vi "Robot Global Data.vi"() -> ()   [LabVIEW 2017]
doc: "This global VI can contain as many global variables as you need. Place a control on the panel, give it a good name. To read or write to it from a VI, drag the icon to the diagram of that VI. You can also drag from the project. Click on the node to change which global you access. You shouldn't have multiple locations writing to a global or it will cause a race-condition."
uses:
  <vilib>/Rock Robotics/WPI/Camera/WPI_CameraImageSize.ctl
  <vilib>/Rock Robotics/WPI/DriverStation/WPI_DriverStationRobotMode2.ctl
panel:
  in  "MotionProfilePos_Right":dbl
  in  "MotionProfilePos_Left":dbl
  in  "Left Drive Position":dbl
  in  "Right Drive Position":dbl
  in  "AutoSwitch":bool
  in  "Record Auto?":bool
  in  "Left Drive Speed":dbl
  in  "Right Drive Speed":dbl
  in  "pistonLock":bool
  in  "MotionProfileVel_Right":dbl
  in  "MotionProfileVel_Left":dbl
  in  "rightEncoder":i32
  in  "leftEncoder":i32
  in  "desiredAngle":dbl
  out "resetEncoder":bool
  in  "distanceInCounts":dbl
  in  "driveStraightSpeed":dbl
  in  "navXYaw":dbl
  in  "leftButtons":bool[](array[boolean])
  in  "manualFirst":bool
  in  "2slide":dbl
  out "secondBottom":bool
  out "secondTop":bool
  out "firstBottom":bool
  out "firstTop":bool
  in  "clawOut":bool
  in  "clawIn":bool
  in  "clawOpen":bool
  in  "clawUp":bool
  in  "driveModes":T1(ring)
  out "rightDrivePower":dbl
  out "leftDrivePower":dbl
  in  "1Sslide":dbl
  in  "Robot Mode":T2
  in  "image size":T3=enum."320x240"
  in  "Enable Vision":bool
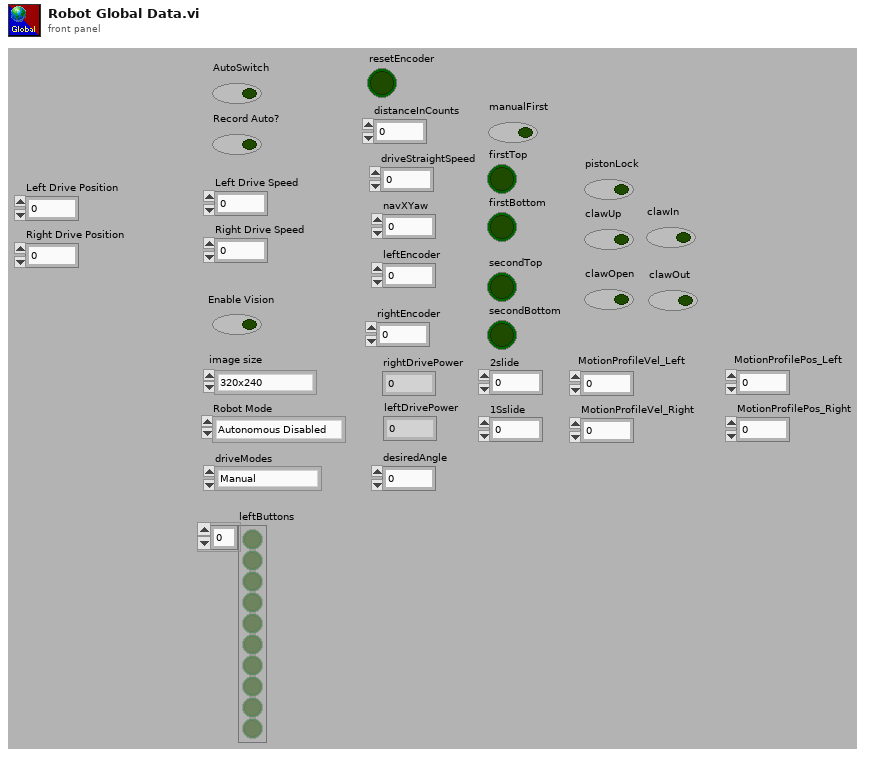
[diagram p1: front panel]
types:
  T1 = enum16{"Manual", "Turn For Angle", "Drive For Distance", "Motion Profile", "Recorded Auto File"}
  T2 = typedef "WPI_DriverStationRobotMode2.ctl" = enum16{"Autonomous Disabled", "Autonomous Enabled", "Teleop Disabled", "Teleop Enabled", "Disconnected", "Finish", "Test Disabled", "Test Enabled", "Emergency Stopped"}
  T3 = typedef "WPI_CameraImageSize.ctl" = enum16{"640x480", "320x240", "160x120", "Custom"}
diagram:
